vi "Read.vi"(0 "System Interface in":refnum<class "System Interface.lvclass">, 11 "Error In":errorcluster) -> (4 "System Interface out":refnum<class "System Interface.lvclass">, 6 "Process Data":T1, 15 "Error Out":errorcluster)   [LabVIEW 2020, in "Boolean.lvlib"]
uses:
  <vilib>/ADAS Record/CustomDataTypes/Boolean/Boolean.lvlib
  <vilib>/ADAS Record/CustomDataTypes/Boolean/Process Data.ctl
  4520f411-daba-4182-bc35-841ea590f987.vi
  <vilib>/FlexLogger/SDK/PluginSDK.lvlibp/PEFClasses/SDK/System Interface/System Interface.lvclass
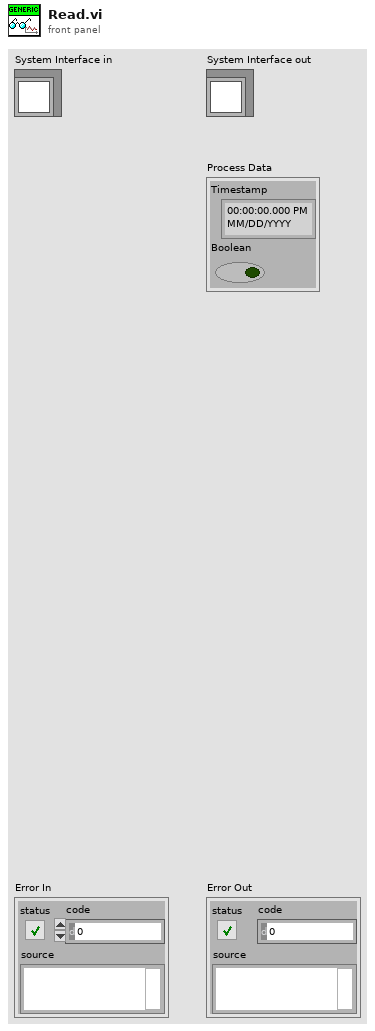
[diagram p1: front panel]
types:
  T1 = typedef "Boolean.lvlib/Process Data.ctl" = cluster{"Timestamp":timestamp, "Boolean":bool}
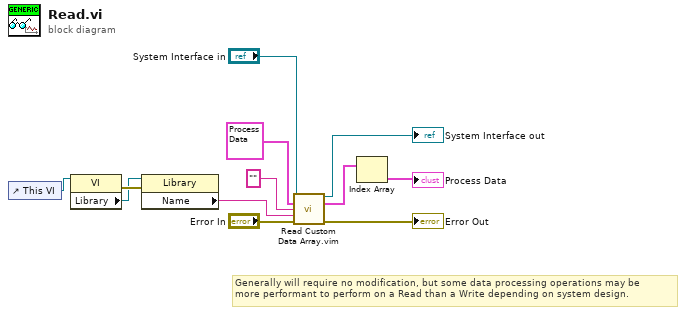
[diagram p0: block diagram]
diagram:
  # "Generally will require no modification, but some data processing operations may be\nmore performant to perform on a Read than a Write depending on system design."
  n1 = control-ref of="This VI"() -> (w4:refnum<vi>)
  n2 = property class="VI"(reference=w4) -> (error out=w3:errorcluster, "Library"=w2:refnum<vi>)  [unwired: 1 in, 1 out]
  n3 = property class="Library"(reference=w2, error in=w3) -> ("Name"=w1:string)  [unwired: 2 out]
  n4 = call "Read Custom Data Array.vim"("System Interface"="System Interface in", "Data Element Type"=T1 {"Timestamp"=timestamp(0 s since 1904-01-01), "Boolean"=FALSE} ("Process Data"), "Metadata Element Type"="" ("appended array"), "Type"=w1, "error in (no error)"="Error In") -> ("System Interface out"=→"System Interface out":refnum<class "System Interface.lvclass">, "Data Array"=w5:T1[], "error out"=→"Error Out":errorcluster)  [unwired: 4 in, 4 out]
  n5 = Index Array(array=w5) -> (element=→"Process Data":T1)  [unwired: 1 in]
